vi "loadRfData.vi"(8 "error in (no error)":errorcluster, 10 "rf":refnum<class "rf.lvclass">, 11 "rfAction in":refnum<class "rfAction.lvclass">) -> (0 "error out":errorcluster, 2 "rf out":refnum<class "rf.lvclass">, 3 "rfAction out":refnum<class "rfAction.lvclass">)   [LabVIEW 2009, in "Views.lvlib" / "ScriptEditor.lvlib" / "rfAction.lvclass"]
uses:
  rfAction.lvclass
  Tools/Scripting/ScriptingEvent/ScriptEvents/Rf Event/rf.lvclass
  rfAction.lvclass/rfAction.ctl
  Tools/DatabaseHelpers/Database Objects/Channel/Channel.lvclass
  Tools/Scripting/ScriptingEvent/ScriptEvents/RfArray/rfArray.lvclass
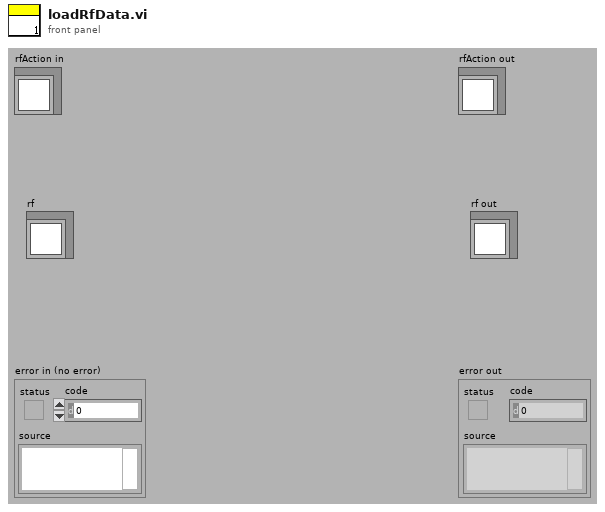
[diagram p1: front panel]
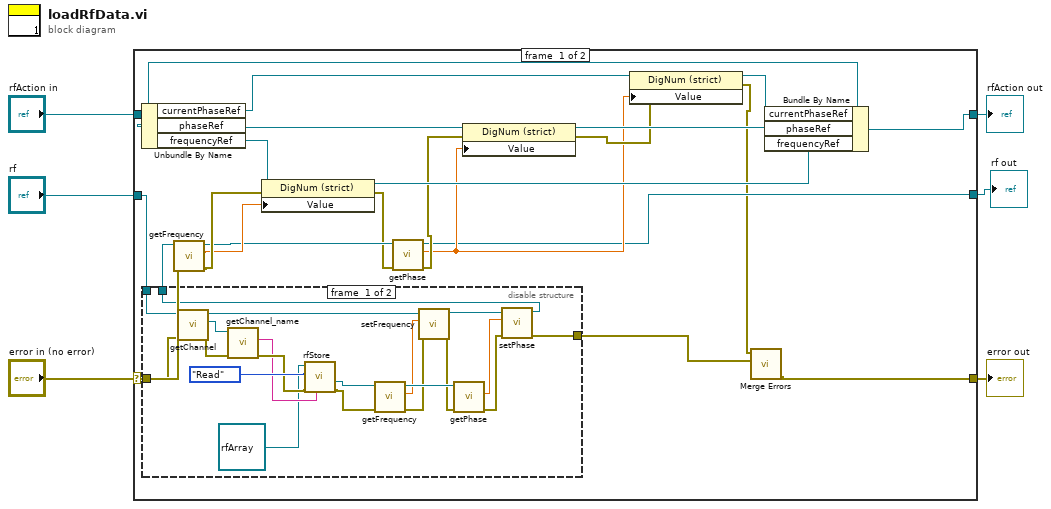
[diagram p0: block diagram]
diagram:
  n1 = case shown="No Error" "error in (no error)" {
    selector: "error in (no error)" -> [w12 w52]
    tunnel: [w11 w52] -> w5
    tunnel: [w27 w51] -> w3
    tunnel: "rfAction in" -> [w28 w51]
    tunnel: "rf" -> [w8 _]
    tunnel: [w13 _] -> w1
    frame #0 {
      n2 = Unbundle By Name(w28) -> ("currentPhaseRef"=w21:refnum<vi>, "phaseRef"=w24:refnum<vi>, "frequencyRef"=w26:refnum<vi>)
      n3 = disable-structure shown="Enabled" {
        disable-tunnel: w12 -> [w39 w50]
        disable-tunnel: [w38 w50] -> w9
        disable-tunnel: w8 -> [w30 w49]
        disable-tunnel: [w29 w49] -> w7
        frame #0 {
          n4 = call-dynamic "getChannel.vi"("error in (no error)"=w39, "ScriptEvent.lvclass in"=w30) -> ("error out"=w40:errorcluster, "Channel.lvclass"=w48:refnum<class "Channel.lvclass">, "ScriptEvent.lvclass out"=w46:refnum<class "rf.lvclass">)  [unwired: 7 in]
          n5 = call "getChannel_name.vi"("error in (no error)"=w40, "Channel.lvclass in"=w48) -> ("error out"=w35:errorcluster, "channel_name"=w34:string)  [unwired: 7 in, 1 out]
          n6 = call "rfStore.vi"("channel_name"=w34, "error in (no error)"=w35, "action"=enum16{"Write", "Read"}."Read", "rfArray in"=refnum<class "rfArray.lvclass"> refnum ("Tools.lvlib:Scripting.lvlib:rfArray.lvclass")) -> ("error out"=w33:errorcluster, "rf out"=w32:refnum<class "rf.lvclass">)  [unwired: 4 in, 2 out]
          n7 = call "getFrequency.vi"("error in (no error)"=w33, "rf in"=w32) -> ("error out"=w45:errorcluster, "frequency"=w44:dbl, "rf out"=w47:refnum<class "rf.lvclass">)  [unwired: 7 in]
          n8 = call "setFrequency.vi"("error in (no error)"=w45, "frequency"=w44, "rf in"=w46) -> ("error out"=w37:errorcluster, "rf out"=w43:refnum<class "rf.lvclass">)  [unwired: 7 in]
          n9 = call "getPhase.vi"("error in (no error)"=w37, "rf in"=w47) -> ("error out"=w41:errorcluster, "phase"=w42:dbl)  [unwired: 7 in, 1 out]
          n10 = call "setPhase.vi"("error in (no error)"=w41, "phase"=w42, "rf in"=w43) -> ("error out"=w38:errorcluster, "rf out"=w29:refnum<class "rf.lvclass">)  [unwired: 7 in]
        }
        frame #1 {
        }
      }
      n11 = call "getFrequency.vi"("error in (no error)"=w12, "rf in"=w7) -> ("error out"=w19:errorcluster, "frequency"=w18:dbl, "rf out"=w17:refnum<class "rf.lvclass">)  [unwired: 7 in]
      n12 = property class="DigNum (strict)"(reference=w26, error in=w19, "Value"=w18) -> (reference out=w25:refnum<vi>, error out=w16:errorcluster)
      n13 = call "getPhase.vi"("error in (no error)"=w16, "rf in"=w17) -> ("error out"=w15:errorcluster, "phase"=w14:dbl, "rf out"=w13:refnum<class "rf.lvclass">)  [unwired: 7 in]
      n14 = property class="DigNum (strict)"(reference=w24, error in=w15, "Value"=w14) -> (reference out=w23:refnum<vi>, error out=w22:errorcluster)
      n15 = property class="DigNum (strict)"(reference=w21, error in=w22, "Value"=w14) -> (reference out=w20:refnum<vi>, error out=w10:errorcluster)
      n16 = call <vilib>:"Merge Errors.vi"("error in 2 (no error)"=w9, "error in 1 (no error)"=w10) -> ("error out"=w11:errorcluster)  [unwired: 5 in]
      n17 = Bundle By Name(cluster=w28, "currentPhaseRef"=w20, "phaseRef"=w23, "frequencyRef"=w25) -> (w27:refnum<class "rfAction.lvclass">)
    }
    frame #1 {
    }
  }
  "error out" <- w5
  "rfAction out" <- w3
  "rf out" <- w1
